vi "RP ADC to Volts element.vi"(6 "osc_fpga_cnv_cnt_to_v method":bool, 7 "Max Volts":sgl=1.0, 11 "ADC data":i16) -> (3 "Volts":sgl format="%_10g")   [LabVIEW 2015]
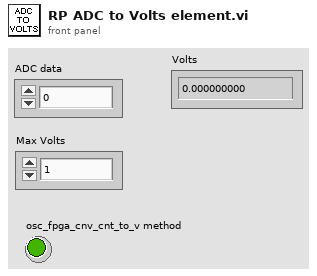
[diagram p1: front panel]
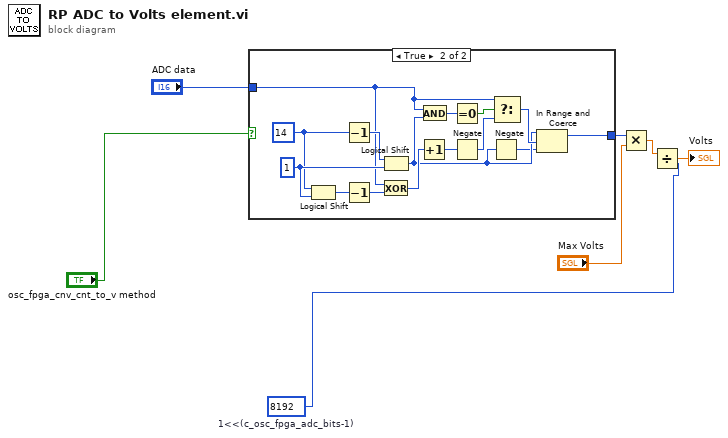
[diagram p0: block diagram]
diagram:
  w2 = 8192  # 1<<(c_osc_fpga_adc_bits-1)
  n1 = case shown="True" "osc_fpga_cnv_cnt_to_v method" {
    tunnel: "ADC data" -> [w8 w13]
    tunnel: [w8 w11] -> w3
    frame False {
    }
    frame True {
      w21 = i16 1
      w18 = i16 14
      n2 = Logical Shift(y=w18, x=w21) -> (x << y=w19:i16)
      n3 = Decrement(x=w18) -> (x-1=w22:i16)
      n4 = Decrement(x=w19) -> (x-1=w20:i16)
      n5 = Logical Shift(y=w22, x=w21) -> (x << y=w10:i16)
      n6 = Exclusive Or(1:w20, 2:w13) -> (0:w16:i16)
      n7 = Increment(x=w16) -> (x+1=w15:i16)
      n8 = And(x=w13, y=w10) -> (x .and. y?=w23:i16)
      n9 = Equal To 0?(x=w23) -> (x = 0?=w17:bool)
      n10 = Negate(x=w15) -> (-x=w14:i16)
      n11 = Negate(x=w10) -> (-x=w9:i16)
      n12 = Select(t=w13, s=w17, f=w14) -> (s? t:f=w12:i16)
      n13 = In Range and Coerce(upper limit=w10, x=w12, lower limit=w9) -> (coerced(x)=w11:i16)  [unwired: 1 out]
    }
  }
  n14 = Multiply(x=w3, y="Max Volts") -> (x*y=w5:sgl)
  n15 = Divide(x=w5, y=w2) -> (x/y=→"Volts":sgl)
